vi "Notify Action Done.vi"(8 "error in (no error)":errorcluster, 11 "Action done":T1) -> (0 "error out":errorcluster)   [LabVIEW 2015]
uses:
  Action/Action Name.ctl
  lib/Sprocket.lvlib
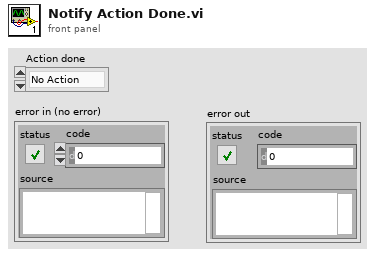
[diagram p1: front panel]
types:
  T1 = typedef "Sprocket.lvlib/Action Name.ctl" = enum16{"No Action", "Drive Left", "Drive Right"}
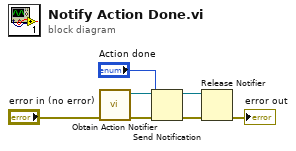
[diagram p0: block diagram]
diagram:
  n1 = call "Obtain Action Notifier.vi"("error in (no error)"="error in (no error)") -> ("error out"=w5:errorcluster, "notifier out"=w1:refnum<notifier>)  [unwired: 9 in]
  n2 = Send Notification(notification="Action done", notifier=w1, error in (no error)=w5) -> (notifier out=w7:refnum<notifier>, error out=w6:errorcluster)
  n3 = Release Notifier(notifier=w7, error in (no error)=w6) -> (error out=→"error out":errorcluster)  [unwired: 1 in, 2 out]
